vi "aft_Simulate_Fixed-Point_FIR_LMS_Configure_Dialog.vi"(11 "State In":T2) -> (2 "Reconfigured?":bool, 3 "State Out":T2)   [LabVIEW 2017, in "NI_AdaptiveFilter.lvlib"]
uses:
  <vilib>/addons/Adaptive Filters/NI_AdaptiveFilter.lvlib
  <vilib>/addons/Adaptive Filters/Utilities/AFT Fixed-Point Settings.ctl
  <vilib>/addons/Adaptive Filters/Fixed-Point Simulation/LMS/AFT Simulate Fixed-Point FIR LMS.ctl
  <vilib>/addons/Adaptive Filters/Utilities/AFT Algorithm.ctl
  <vilib>/addons/Adaptive Filters/Fixed-Point Simulation/LMS/AFT Simulate Fixed-Point FIR LMS.xnode
panel:
  in  "dummy AFT fixed-point settings":T1={"algorithm"=0, "filter length"=128, "step size"=0.0999985, "encoding"={"x(n) word length"=24, "x(n) integer word length"=1, "d(n) word length"=24, "d(n) integer word length"=1, "w(n) word length"=24, "w(n) integer word length"=1, "step size word length"=16, "step size integer word length"=-2}} {"algorithm" items=["LMS"]}
  out "Step size minimum":dbl format="%.4g"
  out "w(n) minimum":dbl format="%.4g"
  out "d(n) minimum":dbl format="%.4g"
  out "x(n) minimum":dbl format="%.4g"
  out "Step size delta":dbl format="%.4g"
  out "Step size maximum":dbl format="%.4g"
  in  "Step size integer word length":i32=-2 min=-128 max=128 format="%.0f bits"
  out "Step size word length":i32=16 min=16 max=16 step=1 format="%.0f bits"
  in  "Save FXP Settings":bool
  in  "Step size":dbl=0.00999832 min=0.0 format="%_6g"
  in  "Filter length":i32=128 min=2
  out "w(n) maximum":dbl format="%.4g"
  out "w(n) delta":dbl format="%.4g"
  out "d(n) maximum":dbl format="%.4g"
  out "d(n) delta":dbl format="%.4g"
  out "x(n) delta":dbl format="%.4g"
  out "x(n) maximum":dbl format="%.4g"
  in  "w(n) word length":i32(ring)=24 items=["16 bits"=16, "24 bits"=24]
  in  "d(n) word length":i32=24 min=16 max=32 step=1 format="%.0f bits"
  in  "d(n) integer word length":i32=1 min=-32 max=32 format="%.0f bits"
  in  "x(n) word length":i32=24 min=16 max=32 step=1 format="%.0f bits"
  in  "x(n) integer word length":i32=1 min=-32 max=32 format="%.0f bits"
  in  "w(n) integer word length":i32=1 min=-32 max=32 format="%.0f bits"
  in  "Help":bool
  in  "Cancel":bool
  in  "OK":bool
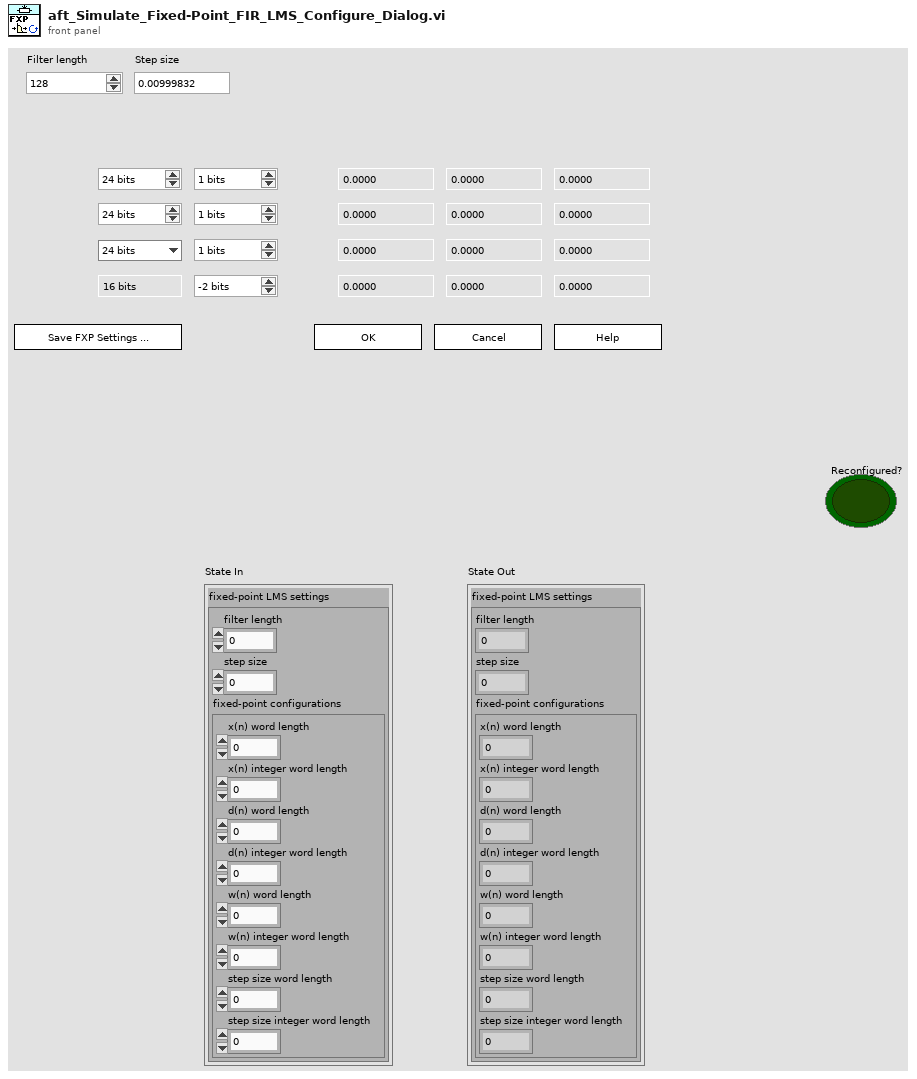
[diagram p1: front panel]
types:
  T1 = typedef "NI_AdaptiveFilter.lvlib/AFT Fixed-Point Settings.ctl" = cluster{"algorithm":u16, "filter length":i32, "step size":dbl, "encoding":cluster{"x(n) word length":i32, "x(n) integer word length":i32, "d(n) word length":i32, "d(n) integer word length":i32, "w(n) word length":i32, "w(n) integer word length":i32, "step size word length":i32, "step size integer word length":i32}}
  T2 = typedef "AFT Simulate Fixed-Point FIR LMS.xnode/AFT Simulate Fixed-Point FIR LMS.ctl" = cluster{"fixed-point LMS settings":cluster{"filter length":i32, "step size":dbl, "fixed-point configurations":cluster{"x(n) word length":i32, "x(n) integer word length":i32, "d(n) word length":i32, "d(n) integer word length":i32, "w(n) word length":i32, "w(n) integer word length":i32, "step size word length":i32, "step size integer word length":i32}}}
  T3 = cluster{"x(n) word length":i32, "x(n) integer word length":i32, "d(n) word length":i32, "d(n) integer word length":i32, "w(n) word length":i32, "w(n) integer word length":i32, "step size word length":i32, "step size integer word length":i32}
  T4 = cluster{"x(n) min":dbl, "d(n) min":dbl, "w(n) min":dbl, "step size min":dbl}
  T5 = cluster{"x(n) max":dbl, "d(n) max":dbl, "w(n) max":dbl, "step size max":dbl}
  T6 = cluster{"x(n) word length":i32, "x(n) integer word length":i32, "d(n) word length":i32, "d(n) integer word length":i32, "w(n) word length":i32, "w(n) integer word length":i32, "Step size word length":i32, "Step size integer word length":i32}
  T7 = typedef "NI_AdaptiveFilter.lvlib/AFT Algorithm.ctl" = u16
  T8 = cluster{"x(n) word length":i32, "x(n) integer word length":i32, "d(n) word length":i32, "d(n) integer word length":i32, "w(n) word length":i32, "w(n) integer word length":i32, i16, "Step size integer word length":i32}
  T9 = cluster{"Filter length":i32, "Step size":dbl, cluster{"x(n) word length":i32, "x(n) integer word length":i32, "d(n) word length":i32, "d(n) integer word length":i32, "w(n) word length":i32, "w(n) integer word length":i32, i16, "Step size integer word length":i32}}
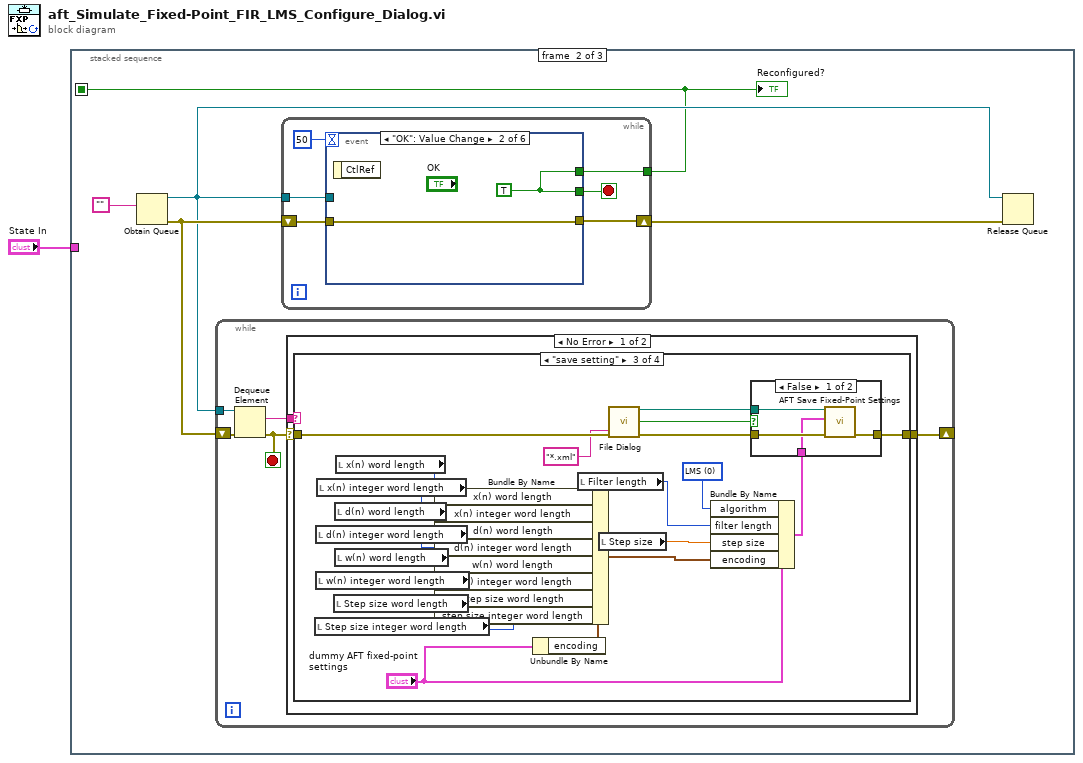
[diagram p0: block diagram]
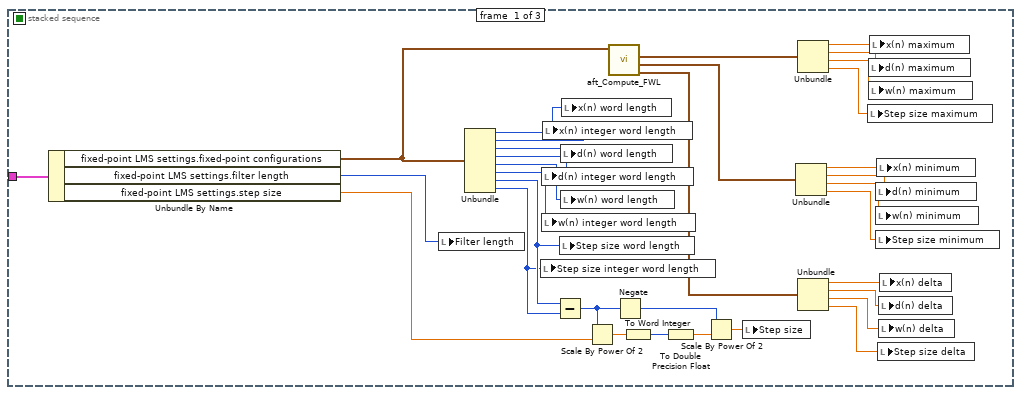
[diagram p2: hidden frame]
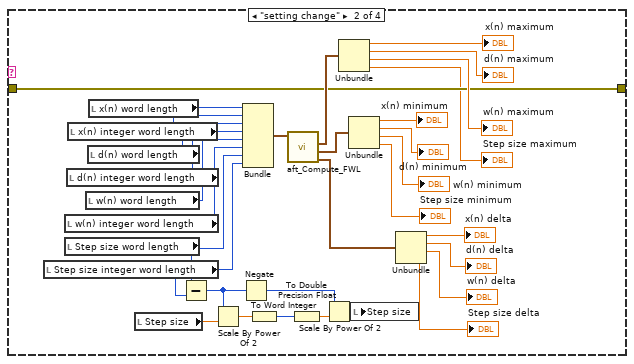
[diagram p4: hidden frame]
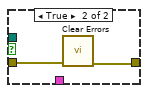
[diagram p5: hidden frame]
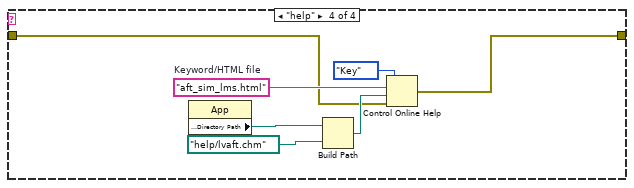
[diagram p6: hidden frame]
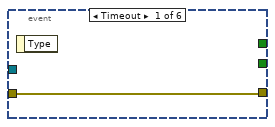
[diagram p8: hidden frame]
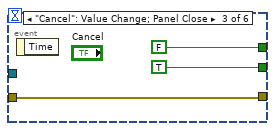
[diagram p9: hidden frame]
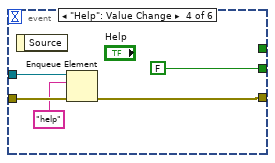
[diagram p10: hidden frame]
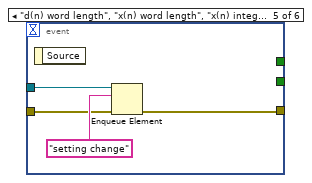
[diagram p11: hidden frame]
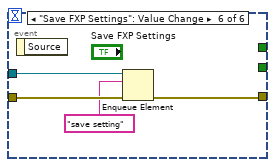
[diagram p12: hidden frame]
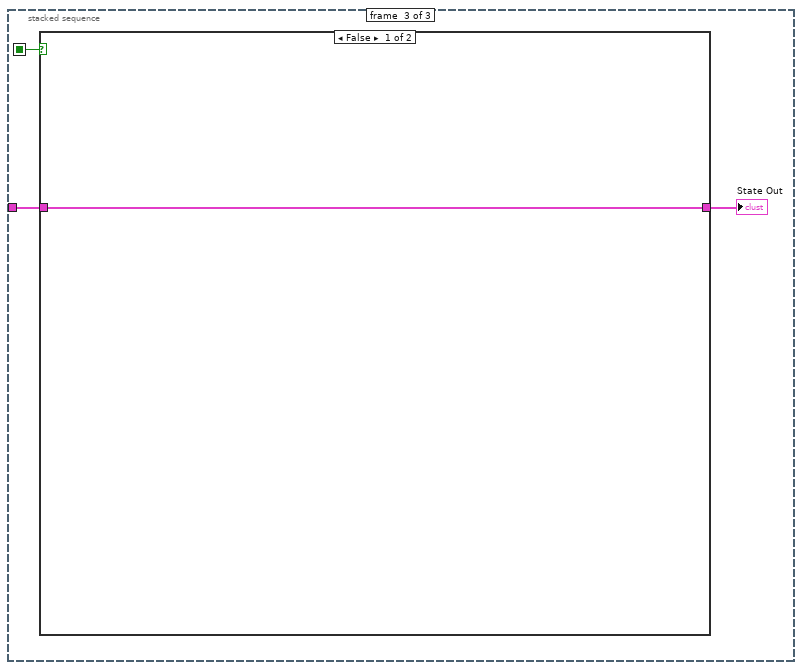
[diagram p13: hidden frame]
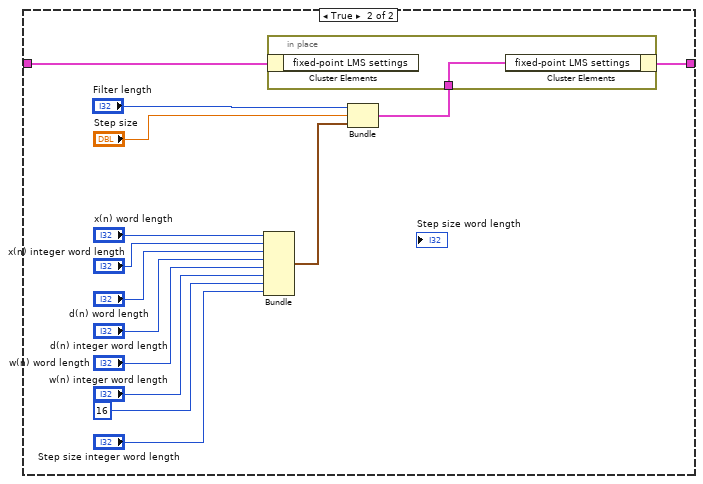
[diagram p14: hidden frame]
diagram:
  n1 = stacked-sequence {
    seq-local: [_ w36 _] -> [_ _ w143]
    tunnel: "State In" -> [w28 _ w142]
    frame #0 {
      n2 = Unbundle By Name(w28) -> ("fixed-point LMS settings.fixed-point configurations"=w20:T3, "fixed-point LMS settings.filter length"=w29:i32, "fixed-point LMS settings.step size"=w11:dbl)
      n3 = local write "Filter length"(w29) -> ()
      n4 = Unbundle(w20) -> ("x(n) word length"=w34:i32, "x(n) integer word length"=w33:i32, "d(n) word length"=w32:i32, "d(n) integer word length"=w31:i32, "w(n) word length"=w30:i32, "w(n) integer word length"=w10:i32, "step size word length"=w9:i32, "step size integer word length"=w8:i32)
      n5 = local write "Step size integer word length"(w8) -> ()
      n6 = local write "d(n) integer word length"(w31) -> ()
      n7 = local write "w(n) integer word length"(w10) -> ()
      n8 = local write "x(n) integer word length"(w33) -> ()
      n9 = Subtract(x=w9, y=w8) -> (x-y=w14:i32)
      n10 = local write "Step size word length"(w9) -> ()
      n11 = local write "d(n) word length"(w32) -> ()
      n12 = local write "w(n) word length"(w30) -> ()
      n13 = local write "x(n) word length"(w34) -> ()
      n14 = Scale By Power Of 2(n=w14, x=w11) -> (x*2^n=w17:dbl)
      n15 = call <vilib>:"aft_Compute_FWL.vi"("fixed-point configurations"=w20) -> ("delta"=w7:cluster{dbl, dbl, dbl, dbl}, "min"=w6:T4, "max"=w27:T5)  [unwired: 8 out]
      n16 = Negate(x=w14) -> (-x=w13:i32)
      n17 = To Word Integer(number=w17) -> (16bit integer=w16:i16)
      n18 = To Double Precision Float(number=w16) -> (double precision float=w15:dbl)
      n19 = Scale By Power Of 2(n=w13, x=w15) -> (x*2^n=w12:dbl)
      n20 = local write "Step size"(w12) -> ()
      n21 = Unbundle(w6) -> ("x(n) min"=w5:dbl, "d(n) min"=w4:dbl, "w(n) min"=w3:dbl, "step size min"=w2:dbl)
      n22 = Unbundle(w27) -> ("x(n) max"=w26:dbl, "d(n) max"=w25:dbl, "w(n) max"=w24:dbl, "step size max"=w18:dbl)
      n23 = Unbundle(w7) -> (w23:dbl, w22:dbl, w21:dbl, w19:dbl)
      n24 = local write "Step size maximum"(w18) -> ()
      n25 = local write "d(n) maximum"(w25) -> ()
      n26 = local write "w(n) maximum"(w24) -> ()
      n27 = local write "x(n) maximum"(w26) -> ()
      n28 = local write "d(n) minimum"(w4) -> ()
      n29 = local write "w(n) minimum"(w3) -> ()
      n30 = local write "Step size minimum"(w2) -> ()
      n31 = local write "x(n) minimum"(w5) -> ()
      n32 = local write "Step size delta"(w19) -> ()
      n33 = local write "d(n) delta"(w22) -> ()
      n34 = local write "w(n) delta"(w21) -> ()
      n35 = local write "x(n) delta"(w23) -> ()
    }
    frame #1 {
      n36 = Obtain Queue(element data type="") -> (queue out=w37:refnum<queue>, error out=w38:errorcluster)  [unwired: 3 in, 2 out]
      n37 = while {
        tunnel: w37 -> [w44]
        shift-right: [w41] -> _
        shift-left: w38 -> [w42]
        stop <- w40 stop-if-true
        n38 = Dequeue Element(queue=w44, error in (no error)=w42) -> (element=w43:string, error out=w40:errorcluster)  [unwired: 3 out]
        n39 = case shown="No Error" w40 {
          selector: w40 -> [w46 w115]
          tunnel: w43 -> [w47 _]
          tunnel: [w45 w115] -> w41
          frame No Error {
            n40 = case shown="\"save setting\"" w47 {
              tunnel: [w48 w73 w101 w109] -> w45
              tunnel: w46 -> [w48 w73 w100 w108]
              frame Default {
              }
              frame "setting change" {
                n41 = local read "Step size integer word length"() -> (w56:i32)
                n42 = local read "w(n) integer word length"() -> (w58:i32)
                n43 = local read "Step size word length"() -> (w57:i32)
                n44 = local read "d(n) integer word length"() -> (w60:i32)
                n45 = local read "x(n) integer word length"() -> (w62:i32)
                n46 = local read "w(n) word length"() -> (w59:i32)
                n47 = local read "d(n) word length"() -> (w61:i32)
                n48 = local read "x(n) word length"() -> (w63:i32)
                n49 = local read "Step size"() -> (w70:dbl)
                n50 = Subtract(x=w57, y=w56) -> (x-y=w66:i32)
                n51 = Scale By Power Of 2(n=w66, x=w70) -> (x*2^n=w69:dbl)
                n52 = Negate(x=w66) -> (-x=w65:i32)
                n53 = Bundle("x(n) word length"=w63, "x(n) integer word length"=w62, "d(n) word length"=w61, "d(n) integer word length"=w60, "w(n) word length"=w59, "w(n) integer word length"=w58, "Step size word length"=w57, "Step size integer word length"=w56) -> (w55:T6)  [unwired: 1 out]
                n54 = To Word Integer(number=w69) -> (16bit integer=w68:i16)
                n55 = call <vilib>:"aft_Compute_FWL.vi"("fixed-point configurations"=w55) -> ("delta"=w54:cluster{dbl, dbl, dbl, dbl}, "min"=w53:T4, "max"=w80:T5)  [unwired: 8 out]
                n56 = To Double Precision Float(number=w68) -> (double precision float=w67:dbl)
                n57 = Scale By Power Of 2(n=w65, x=w67) -> (x*2^n=w64:dbl)
                n58 = Unbundle(w80) -> ("x(n) max"=→"x(n) maximum":dbl, "d(n) max"=→"d(n) maximum":dbl, "w(n) max"=→"w(n) maximum":dbl, "step size max"=→"Step size maximum":dbl)
                n59 = Unbundle(w53) -> ("x(n) min"=→"x(n) minimum":dbl, "d(n) min"=→"d(n) minimum":dbl, "w(n) min"=→"w(n) minimum":dbl, "step size min"=→"Step size minimum":dbl)
                n60 = local write "Step size"(w64) -> ()
                n61 = Unbundle(w54) -> (→"x(n) delta":dbl, →"d(n) delta":dbl, →"w(n) delta":dbl, →"Step size delta":dbl)
              }
              frame "save setting" {
                w81 = T7 0 items=["LMS"] ("algorithm")
                n62 = local read "Step size integer word length"() -> (w83:i32)
                n63 = local read "d(n) integer word length"() -> (w88:i32)
                n64 = local read "w(n) integer word length"() -> (w86:i32)
                n65 = local read "x(n) integer word length"() -> (w90:i32)
                n66 = local read "Step size word length"() -> (w84:i32)
                n67 = local read "d(n) word length"() -> (w89:i32)
                n68 = local read "w(n) word length"() -> (w87:i32)
                n69 = local read "x(n) word length"() -> (w91:i32)
                n70 = Unbundle By Name("dummy AFT fixed-point settings") -> ("encoding"=w85:T3)
                n71 = Bundle By Name(cluster=w85, "x(n) word length"=w91, "x(n) integer word length"=w90, "d(n) word length"=w89, "d(n) integer word length"=w88, "w(n) word length"=w87, "w(n) integer word length"=w86, "step size word length"=w84, "step size integer word length"=w83) -> (w82:T3)
                n72 = local read "Filter length"() -> (w95:i32)
                n73 = local read "Step size"() -> (w94:dbl)
                n74 = call "File Dialog"("error in"=w100, "pattern (all files)"="*.xml") -> ("selected path"=w97:path, "cancelled"=w98:bool, "error out"=w99:errorcluster)  [unwired: 5 in, 6 out]
                n75 = Bundle By Name(cluster="dummy AFT fixed-point settings", "algorithm"=w81, "filter length"=w95, "step size"=w94, "encoding"=w82) -> (w93:T1)
                n76 = case shown="False" w98 {
                  tunnel: [w105 w106] -> w101
                  tunnel: w99 -> [w104 w107]
                  tunnel: w97 -> [w103 _]
                  tunnel: w93 -> [w102 _]
                  frame False {
                    n77 = call <vilib>:"AFT Save Fixed-Point Settings.vi"("error in (no error)"=w104, "fixed-point settings"=w102, "file path in"=w103) -> ("error out"=w105:errorcluster)  [unwired: 8 out]
                  }
                  frame True {
                    n78 = call <vilib>:"Clear Errors.vi"("error in (no error)"=w107) -> ("error out"=w106:errorcluster)  [unwired: 1 in, 5 out]
                  }
                }
              }
              frame "help" {
                w112 = "aft_sim_lms.html"  # Keyword/HTML file
                n79 = property class="App"() -> ("Application:Directory Path"=w114:path)  [unwired: 2 in, 2 out]
                n80 = Build Path(base path=w114, name or relative path=path "help/lvaft.chm") -> (appended path=w111:path)
                n81 = Control Online Help(1:w108, 2:w111, 3:w112, 4:enum16{"Contents", "Key", "Close"}."Key" ("Operation")) -> (0:w109:errorcluster)
              }
            }
          }
          frame Error {
          }
        }
      }
      n82 = while {
        tunnel: w37 -> [w121]
        shift-right: [w118] -> w35
        shift-left: w38 -> [w120]
        tunnel: [w116] -> w36
        stop <- w117 stop-if-true
        n83 = event shown="[1] \"OK\": Value Change" {
          selector: _ -> [_ _ _ _ _ _]
          dyn-events: _ -> [_ _ _ _ _ _]
          timeout: 50 -> [_ _ _ _ _ _]
          tunnel: w121 -> [_ _ _ w131 w135 w140]
          tunnel: w120 -> [w122 w123 w125 w130 w134 w139]
          tunnel: [w122 w123 w125 w129 w133 w138] -> w118
          tunnel: [_ w124 FALSE _ _ _] -> w116
          tunnel: [_ w124 TRUE FALSE _ _] -> w117
          event Timeout {
            n84 = event-data() -> ()  [unwired: 2 out]
          }
          event "OK": Value Change {
            w124 = TRUE
            n85 = event-data() -> ()  [unwired: 2 out]
          }
          event "Cancel": Value Change; Panel Close {
            n86 = event-data() -> ()  [unwired: 2 out]
          }
          event "Help": Value Change {
            n87 = event-data() -> ()  [unwired: 2 out]
            n88 = Enqueue Element(queue=w131, element="help", error in (no error)=w130) -> (error out=w129:errorcluster)  [unwired: 3 out]
          }
          event "d(n) word length", "x(n) word length", "x(n) integer word length", "d(n) integer word length", "w(n) integer word length", "w(n) word length", "Step size word length", "Step size integer word length", "Step size": Value Change {
            n89 = event-data() -> ()  [unwired: 2 out]
            n90 = Enqueue Element(queue=w135, element="setting change", error in (no error)=w134) -> (error out=w133:errorcluster)  [unwired: 3 out]
          }
          event "Save FXP Settings": Value Change {
            n91 = event-data() -> ()  [unwired: 2 out]
            n92 = Enqueue Element(queue=w140, element="save setting", error in (no error)=w139) -> (error out=w138:errorcluster)  [unwired: 3 out]
          }
        }
      }
      "Reconfigured?" <- w36
      n93 = Release Queue(queue=w37, error in (no error)=w35) -> ()  [unwired: 4 out]
    }
    frame #2 {
      n94 = case shown="False" w143 {
        tunnel: w142 -> [w144 w156]
        tunnel: [w144 w154] -> w141
        frame False {
        }
        frame True {
          n95 = Bundle("x(n) word length"="x(n) word length", "x(n) integer word length"="x(n) integer word length", "d(n) word length"="d(n) word length", "d(n) integer word length"="d(n) integer word length", "w(n) word length"="w(n) word length", "w(n) integer word length"="w(n) integer word length", i16 16, "Step size integer word length"="Step size integer word length") -> (w145:T8)  [unwired: 1 out]
          n96 = Bundle("Filter length"="Filter length", "Step size"="Step size", w145) -> (w155:T9)  [unwired: 1 out]
          n97 = in-place {
            in-place-border: w155 -> [w159]
            n98 = in-place-cluster #1(w156) -> ()  [unwired: 1 out]
            n99 = in-place-cluster #1("fixed-point LMS settings"=w159) -> (w154:T2)
          }
        }
      }
      "State Out" <- w141
    }
  }
